vi "WD_AS_Update_database.vi"(7 "計算用array":cluster{"條碼A":string, "條碼B":string}[](array[cluster])=[{"條碼A"="", "條碼B"="80540"}, {"條碼A"="7834", "條碼B"="80540"}, {"條碼A"="453", "條碼B"="453"}], 8 "error in (no error)":errorcluster, 9 "站點總數":i32=5, 10 "當前料數":i32=2, 11 "DBLink":string="Driver={ODBC Driver 17 for SQL Server};Server=localhost\\SQLEXPRESS;Database=ZDX201;UID=labview;PWD=Dsa@54137926") -> (0 "error out":errorcluster)   [LabVIEW 2019]
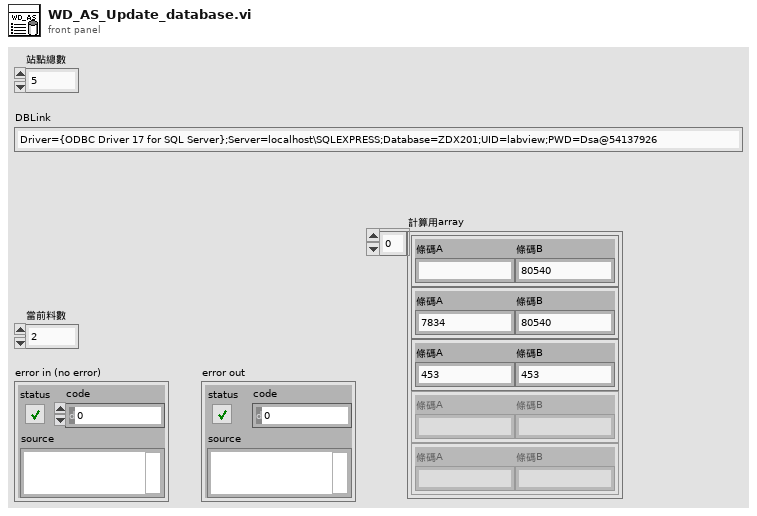
[diagram p1: front panel]
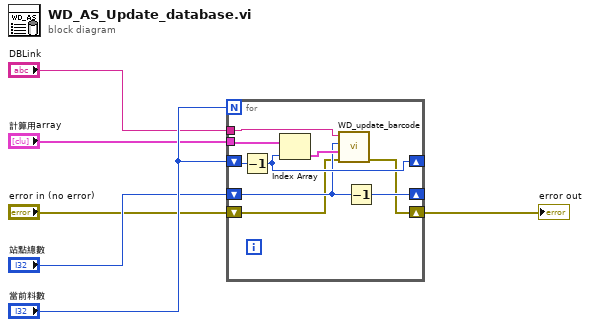
[diagram p0: block diagram]
diagram:
  n1 = for {
    N: "當前料數" -> [_]
    shift-right: [w7] -> w2
    shift-left: "error in (no error)" -> [w8]
    tunnel: "計算用array" -> [w15]
    shift-right: [w11] -> _
    shift-left: "當前料數" -> [w14]
    tunnel: "DBLink" -> [w12]
    shift-right: [w10] -> _
    shift-left: "站點總數" -> [w9]
    n2 = Decrement(x=w14) -> (x-1=w11:i32)
    n3 = Index Array(array=w15, index=w11) -> (element=w13:cluster{"條碼A":string, "條碼B":string})
    n4 = call "WD_update_barcode.vi"("error in (no error)"=w8, "Workplace data"=w13, "workplace_id"=w9, "DBlink"=w12) -> ("error out"=w7:errorcluster)  [unwired: 7 in]
    n5 = Decrement(x=w9) -> (x-1=w10:i32)
  }
  "error out" <- w2
